vi "Test_LaunchAndCloseAbstractFramework_NoError.vi"(8 "error in (no error)":errorcluster, 11 "TestCase in":refnum<class "TestIViewModel.lvclass">) -> (0 "error out":errorcluster, 3 "TestCase out":refnum<class "TestIViewModel.lvclass">)   [LabVIEW 2020, in "TestIViewModel.lvclass"]
uses:
  TestIViewModel.lvclass
  TestIViewModel.lvclass/TestIViewModel.ctl
  Source/IViewModel/IViewModel/IViewModel.lvclass
  Source/IViewable/IViewable/IViewable.lvclass
  modules/mva-core/Source/IModel/IModel/IModel.lvclass
  <vilib>/ActorFramework/Actor/Actor.lvclass
  <vilib>/ActorFramework/Stop Msg/Stop Msg.lvclass
  modules/mva-core/Source/IMediator/IMediator/IMediator.lvclass
  7727fa57-eb30-48e2-80b1-fe3e46426cb7.vi
  C:/Git/mva-viewable/Source/IViewManager/IViewManager/IViewManager.lvclass
  C:/Git/mva-viewable/Source/IViewable/IViewable/IViewable.lvclass
  C:/Git/mva-viewable/Source/ActorEvents/IEventAggregator/IEventAggregator.lvclass
  C:/Git/mva-viewable/modules/mva-core/Source/IObserver/IObserver/IObserver.lvclass
  C:/Program Files (x86)/National Instruments/LabVIEW 2020/vi.lib/ActorFramework/Actor/Actor.lvclass
  C:/Git/mva-viewable/Source/IViewModel/IViewModel/IViewModel.lvclass
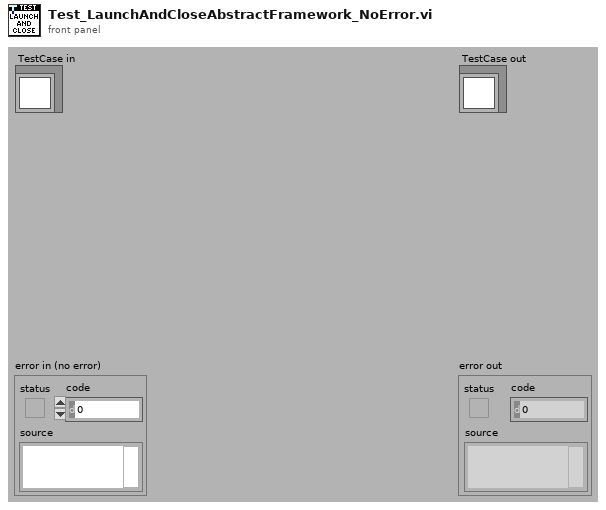
[diagram p1: front panel]
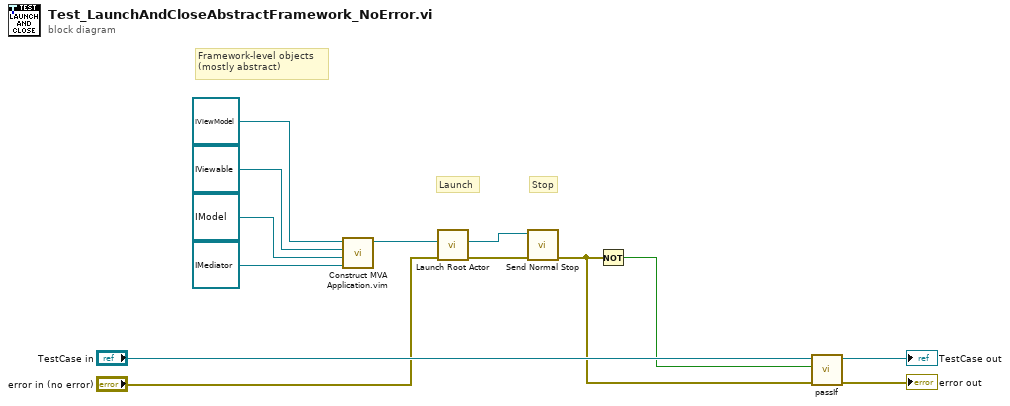
[diagram p0: block diagram]
diagram:
  # "Stop"
  # "Launch"
  # "Framework-level objects\n(mostly abstract)"
  n1 = call "Construct MVA Application.vim"("Mediator Type"=refnum<class "IMediator.lvclass"> refnum ("Mediator"), "Model Type"=refnum<class "IModel.lvclass"> refnum ("Model"), "Startup View Configuration"=refnum<class "IViewable.lvclass"> refnum, "IViewModel In"=refnum<class "IViewModel.lvclass"> refnum) -> ("IViewModel Out"=w5:refnum<class "IViewModel.lvclass">)  [unwired: 7 in]
  n2 = call <vilib>:"Launch Root Actor.vi"("error in (no error)"="error in (no error)", "Actor"=w5) -> ("error out"=w3:errorcluster, "Actor's Enqueuer"=w4:refnum<class "Message Enqueuer.lvclass">)  [unwired: 8 in]
  n3 = call <vilib>:"Send Normal Stop.vi"("error in (no error)"=w3, "Message Enqueuer"=w4) -> ("error out"=w1:errorcluster)  [unwired: 9 in]
  n4 = Not(x=w1) -> (.not. x?=w10:bool)
  n5 = call-dynamic "passIf.vi"("error in (no error)"=w1, "pass"=w10, "TestCase in"="TestCase in") -> ("error out"=→"error out":errorcluster, "TestCase out"=→"TestCase out":refnum<class "TestIViewModel.lvclass">)  [unwired: 7 in]
